vi "FTW-Actor-Construct.vi"(0 "FTW Actor Instance Type":refnum<class "FTW-ActorInstance.lvclass">, 7 "Actor Instance Configuration":string, 11 "error in":errorcluster) -> (4 "FTW Actor Instance":refnum<class "FTW-ActorInstance.lvclass">, 6 "Incoming Requests":refnum<event-registration>, 8 "Local Messages":refnum<event-registration>, 15 "error out":errorcluster)   [LabVIEW 2015, in "FTW-ActorInstance.lvclass"]
uses:
  FTW-ActorInstance.lvclass
  Message/Request/FTW-Message-IncomingRequest.lvclass
  Message/Base/FTW-Message.lvclass
  FTW-ActorInstance.lvclass/FTW-ActorInstance.ctl
  JSON/core/FTW-JSON-Core-EncodingFlags.vi
  JSON/FTW-JSON-Parse.vi
  Reflection/FTW-Reflection-Type.vi
  CodeGen/JSON Deserialize/FTW-JSON-Core-GetFlattenedValue.vi
  CodeGen/JSON Deserialize/FTW-JSON-Deserialize.xnode
  Endpoint/FTW-Endpoint.lvclass
  Ether/FTW-Ether.lvclass
  Reply/FTW-Reply.lvclass
panel:
  # "Inputs"
  # "Outputs"
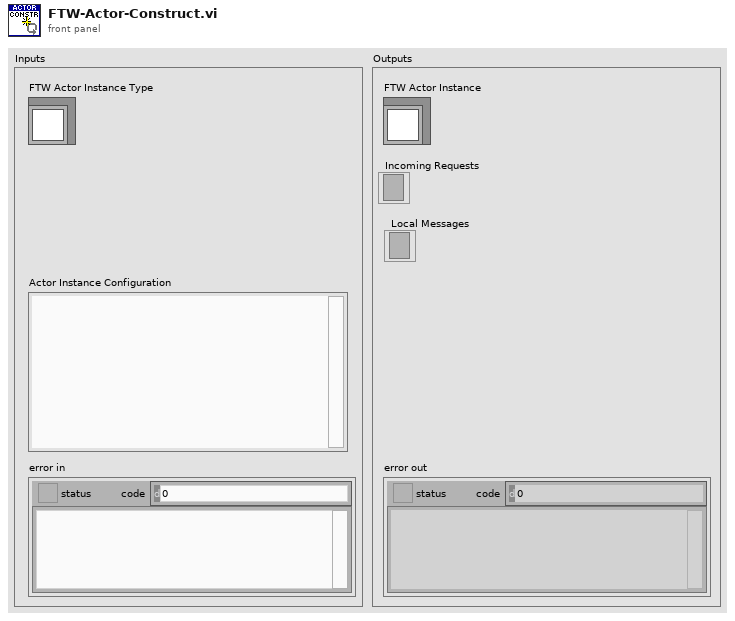
[diagram p1: front panel]
types:
  T1 = cluster{"InboxAddress":string, "LauncherAddress":string}
  T2 = typedef "FTW-MessagePayload.ctl" = cluster{"Header":string, "Body":string, "FTW: Sender Identity":string, "FTW: Reply Address":string, "FTW: Reply Error":errorcluster}
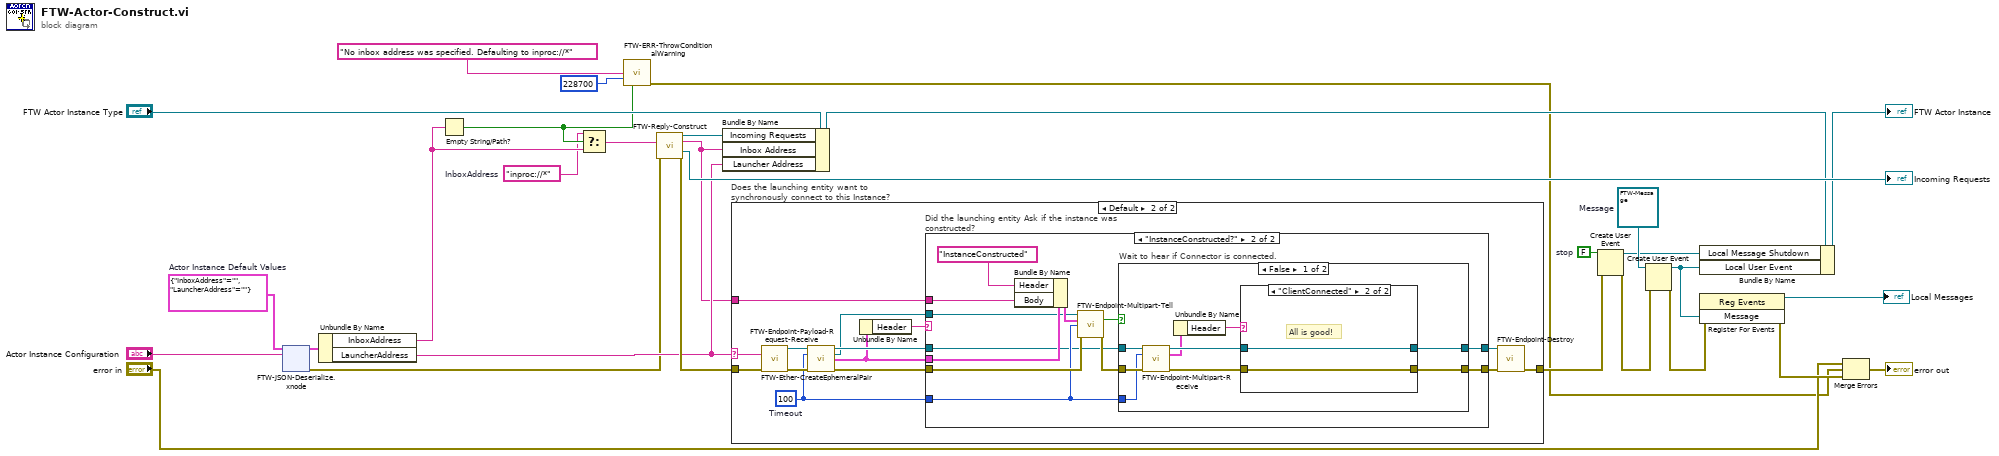
[diagram p0: block diagram]
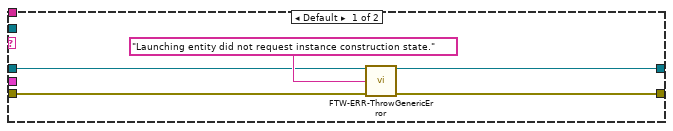
[diagram p3: hidden frame]
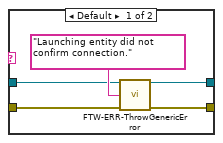
[diagram p4: hidden frame]
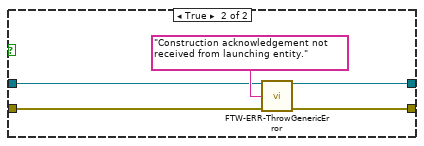
[diagram p5: hidden frame]
diagram:
  w1 = T1 {"InboxAddress"="", "LauncherAddress"=""}  # Actor Instance Default Values
  w2 = "inproc://*"  # InboxAddress
  w17 = FALSE  # stop
  w24 = refnum<class "FTW-Message.lvclass"> refnum  # Message
  n1 = xnode "FTW-JSON-Deserialize.xnode"("Type and Defaults"=w1, "JSON String"="Actor Instance Configuration") -> ("Values"=w25:T1, "error out"=w7:errorcluster)  [unwired: 1 in]
  n2 = Unbundle By Name(w25) -> ("InboxAddress"=w4:string, "LauncherAddress"=w15:string)
  n3 = Empty String/Path?(string/path=w4) -> (empty?=w5:bool)
  n4 = Select(t=w2, s=w5, f=w4) -> (s? t:f=w3:string)
  n5 = call "FTW-ERR-ThrowConditionalWarning.vi"("Warning Message"="No inbox address was specified. Defaulting to inproc://*", "Error Code"=228700, "Throw?"=w5) -> ("error out"=w6:errorcluster)  [unwired: 12 in]
  n6 = call "FTW-Reply-Construct.vi"("Address"=w3, "error in"=w7) -> ("FTW-Router Out"=w14:refnum<class "FTW-Reply.lvclass">, "Actual Address"=w13:string, "Event Registration Refnum"=→"Incoming Requests":refnum<event-registration>, "error out"=w26:errorcluster)  [unwired: 10 in]
  n7 = Bundle By Name(cluster="FTW Actor Instance Type", "Incoming Requests"=w14, "Inbox Address"=w13, "Launcher Address"=w15) -> (w16:refnum<class "FTW-ActorInstance.lvclass">)
  n8 = case "Does the launching entity want to synchronously connect to this Instance?" shown="Default" w15 {
    selector: w15 -> [_ w36]
    tunnel: w26 -> [w31 w38]
    tunnel: w13 -> [_ w45]
    tunnel: [w31 w41] -> w12
    frame "" {
    }
    frame Default {
      w35 = 100  # Timeout
      n9 = call "FTW-Ether-CreateEphemeralPair.vi"("Requested Ephemeral Address"=w36, "error in"=w38) -> ("Ephemeral Endpoint"=w39:refnum<class "FTW-Endpoint.lvclass">, "error out"=w37:errorcluster)  [unwired: 11 in, 1 out]
      n10 = call-dynamic "FTW-Endpoint-Payload-Request-Receive.vi"("FTW Endpoint"=w39, "Timeout"=w35, "error in"=w37) -> ("FTW Endpoint out"=w43:refnum<class "FTW-Endpoint.lvclass">, "Reply Endpoint"=w32:refnum<class "FTW-Endpoint.lvclass">, "Payload"=w33:T2, "error out"=w44:errorcluster)  [unwired: 8 in, 1 out]
      n11 = Unbundle By Name(w33) -> ("Header"=w34:string)
      n12 = case "Did the launching entity Ask if the instance was constructed?" shown="\"InstanceConstructed?\"" w34 {
        tunnel: w45 -> [_ w52]
        tunnel: w44 -> [w49 w61]
        tunnel: w43 -> [w46 w51]
        tunnel: [w48 w59] -> w40
        tunnel: [w46 w57] -> w42
        tunnel: w35 -> [_ w56]
        tunnel: w33 -> [_ w55]
        tunnel: w32 -> [_ w50]
        frame Default {
          n13 = call "FTW-ERR-ThrowGenericError.vi"("Error Message"="Launching entity did not request instance construction state.", "error in"=w49) -> ("error out"=w48:errorcluster)  [unwired: 13 in]
        }
        frame "InstanceConstructed?" {
          n14 = Bundle By Name(cluster=w55, "Header"="InstanceConstructed", "Body"=w52) -> (w54:T2)
          n15 = call-dynamic "FTW-Endpoint-Multipart-Tell.vi"("FTW Endpoint"=w50, "Message"=w54, "Timeout"=w56, "error in"=w61) -> ("Timed out?"=w58:bool, "error out"=w60:errorcluster)  [unwired: 9 in, 1 out]
          n16 = case "Wait to hear if Connector is connected." shown="False" w58 {
            tunnel: w51 -> [w68 w77]
            tunnel: w60 -> [w66 w79]
            tunnel: w56 -> [w65 _]
            tunnel: [w69 w78] -> w59
            tunnel: [w70 w77] -> w57
            frame False {
              n17 = call-dynamic "FTW-Endpoint-Multipart-Receive.vi"("FTW Endpoint"=w68, "Timeout"=w65, "error in"=w66) -> ("FTW Endpoint out"=w67:refnum<class "FTW-Endpoint.lvclass">, "Message Received"=w63:T2, "error out"=w64:errorcluster)  [unwired: 9 in, 1 out]
              n18 = Unbundle By Name(w63) -> ("Header"=w62:string)
              n19 = case shown="\"ClientConnected\"" w62 {
                tunnel: w67 -> [w72 w76]
                tunnel: w64 -> [w73 w75]
                tunnel: [w72 w76] -> w70
                tunnel: [w71 w75] -> w69
                frame Default {
                  n20 = call "FTW-ERR-ThrowGenericError.vi"("Error Message"="Launching entity did not confirm connection.", "error in"=w73) -> ("error out"=w71:errorcluster)  [unwired: 13 in]
                }
                frame "ClientConnected" {
                  # "All is good!"
                }
              }
            }
            frame True {
              n21 = call "FTW-ERR-ThrowGenericError.vi"("Error Message"="Construction acknowledgement not received from launching entity.", "error in"=w79) -> ("error out"=w78:errorcluster)  [unwired: 13 in]
            }
          }
        }
      }
      n22 = call-dynamic "FTW-Endpoint-Destroy.vi"("FTW Endpoint"=w42, "error in"=w40) -> ("error out"=w41:errorcluster)  [unwired: 13 in]
    }
  }
  n23 = Create User Event(user event datatype=w17, error in=w12) -> (user event=w18:refnum<user-event>, error out=w19:errorcluster)
  n24 = Create User Event(user event datatype=w24, error in=w19) -> (user event=w20:refnum<user-event>, error out=w23:errorcluster)
  n25 = Bundle By Name(cluster=w16, "Local Message Shutdown"=w18, "Local User Event"=w20) -> (→"FTW Actor Instance":refnum<class "FTW-ActorInstance.lvclass">)
  n26 = register-events(error in=w23, w20) -> (reference out=→"Local Messages":refnum<event-registration>, error out=w21:errorcluster)  [unwired: 1 in]
  n27 = Merge Errors("error in", w6, w21) -> (→"error out":errorcluster)
